vi "LoadConfigFile.vi"(8 "error in":errorcluster, 11 "Model Name":string) -> (0 "error out":errorcluster, 1 "path":path, 2 "ConnectConfig":T1={"IP Address"="", "Port"=102, "Timeout"=5000}, 3 "Data out":T2)   [LabVIEW 2025, in "PLC_Module.lvlib" / "PLC_Module.lvclass"]
uses:
  PLC_Module.lvclass
  PLC_Data_Config.ctl
  PLC_Data.ctl
  PLC_Data_Type.ctl
  PLC_Connect_Config.ctl
  PLC_Config.ctl
  a0ae5e0e-cf4b-4af0-ab00-451458f61aa5.vi
  <vilib>/JDP Science/JSONtext/JSON text to Variant.vi
  <vilib>/JDP Science/JSONtext/LVClass Serializer/JSONtext LVClass Serializer.lvclass
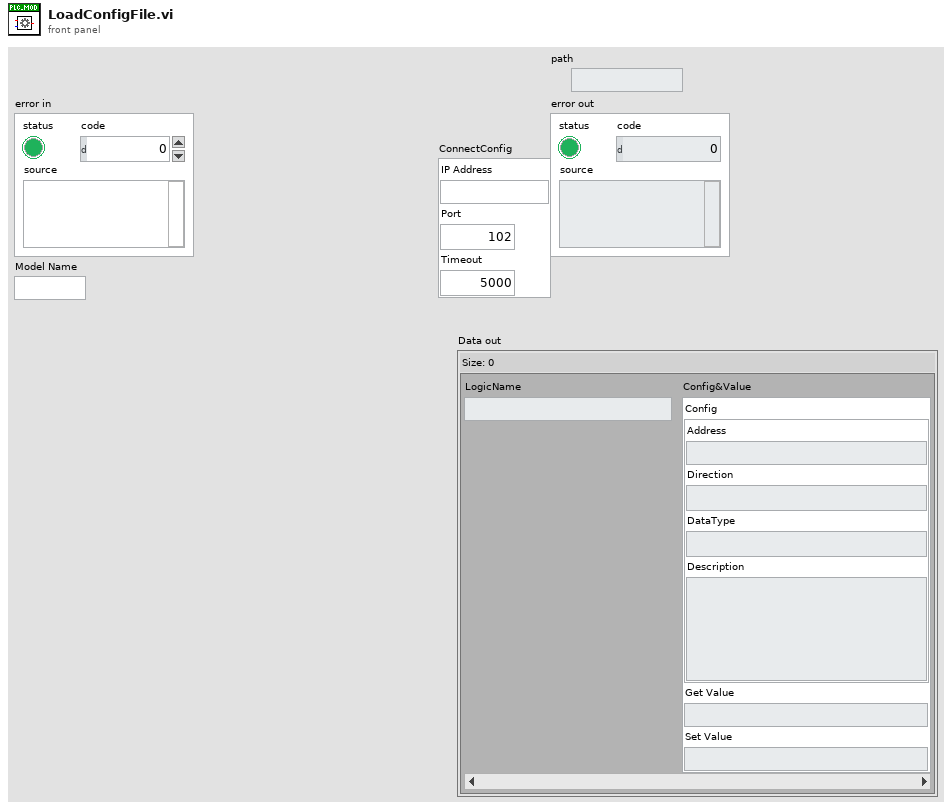
[diagram p1: front panel]
types:
  T1 = typedef "PLC_Module.lvlib/PLC_Module.lvclass/PLC_Connect_Config.ctl" = cluster{"IP Address":string, "Port":u16, "Timeout":i32}
  T2 = typedef "PLC_Module.lvlib/PLC_Module.lvclass/PLC_Data_Config.ctl" = map{string, cluster{"Config":T3, "Get Value":string, "Set Value":string}}
  T3 = typedef "PLC_Module.lvlib/PLC_Module.lvclass/PLC_Data.ctl" = cluster{"Address":string, "Direction":enum16{"PC->PLC", "PLC->PC"}, "DataType":T4, "Description":string}
  T4 = typedef "PLC_Module.lvlib/PLC_Module.lvclass/PLC_Data_Type.ctl" = enum16{"Boolean", "Single Float", "U8", "U32", "U32_Array", "String"}
  T5 = typedef "PLC_Module.lvlib/PLC_Module.lvclass/PLC_Config.ctl" = cluster{"ConnectConfig":T1, "DataConfiguration":T2}
  T6 = enum16{"open", "replace", "create", "open or create", "replace or create", "replace or create with confirmation"}
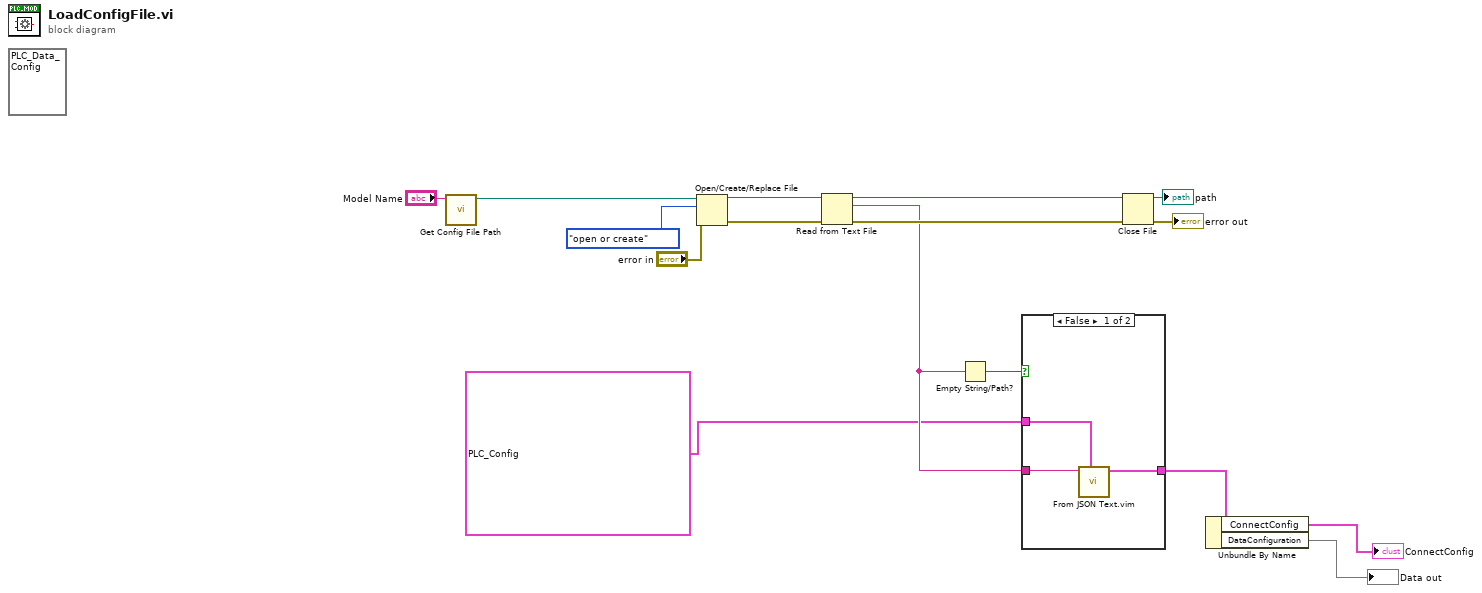
[diagram p0: block diagram]
diagram:
  (unwired) T2 {"PC_AutoManualMode"={"Config"={"Address"="DB6010.703", "Direction"=enum."PC->PLC", "DataType"=enum."U8", "Description"="PC手自动模式"}, "Get Value"="", "Set Value"=""}, "PC_Error"={"Config"={"Address"="DB6010.700[3]", "Direction"=enum."PC->PLC", "DataType"=enum."Boolean", "Description"="错误信息"}, "Get Value"="", "Set Value"=""}, "PC_ErrorCode"={"Config"={"Address"="DB6010.714", "Direction"=enum."PC->PLC", "DataType"=enum."U32", "Description"=""}, "Get Value"="", "Set Value"=""}, "PC_FDBK_1"={"Config"={"Address"="DB6010.704", "Direction"=enum."PC->PLC", "DataType"=enum."U32", "Description"="读取测试流程信号"}, "Get Value"="", "Set Value"=""}, "PC_HeartBeat"={"Config"={"Address"="DB6010.700[0]", "Direction"=enum."PC->PLC", "DataType"=enum."Boolean", "Description"="PC端心跳信号"}, "Get Value"="", "Set Value"=""}, "PC_ProdCode"={"Config"={"Address"="DB6010.750", "Direction"=enum."PC->PLC", "DataType"=enum."U32", "Description"="向PLC发送配方号"}, "Get Value"="", "Set Value"=""}, "PC_ProdName"={"Config"={"Address"="DB6010.720[28]", "Direction"=enum."PC->PLC", "DataType"=enum."String", "Description"="向PLC发送配方名称"}, "Get Value"="", "Set Value"=""}, "PC_Ready"={"Config"={"Address"="DB6010.700[6]", "Direction"=enum."PC->PLC", "DataType"=enum."Boolean", "Description"=""}, "Get Value"="", "Set Value"=""}, "PC_Running"={"Config"={"Address"="DB6010.700[5]", "Direction"=enum."PC->PLC", "DataType"=enum."Boolean", "Description"=""}, "Get Value"="", "Set Value"=""}, "PC_TotleResult"={"Config"={"Address"="DB6012.0", "Direction"=enum."PC->PLC", "DataType"=enum."U32", "Description"="向PLC发送测试总结果"}, "Get Value"="", "Set Value"=""}, "PLC_AutoManualMode"={"Config"={"Address"="DB6010.3", "Direction"=enum."PLC->PC", "DataType"=enum."U8", "Description"="PLC手自动模式"}, "Get Value"="", "Set Value"=""}, "PLC_DMC"={"Config"={"Address"="DB6010.100[48]", "Direction"=enum."PLC->PC", "DataType"=enum."String", "Description"="从PLC读取SN"}, "Get Value"="", "Set Value"=""}, "PLC_HeartBeat"={"Config"={"Address"="DB6010.0[0]", "Direction"=enum."PLC->PC", "DataType"=enum."Boolean", "Description"="PLC端心跳信号"}, "Get Value"="", "Set Value"=""}, "PLC_ProdCode"={"Config"={"Address"="DB6010.70", "Direction"=enum."PLC->PC", "DataType"=enum."U32", "Description"="向PC发送交互信号"}, "Get Value"="", "Set Value"=""}, "PLC_ProdName"={"Config"={"Address"="DB6010.40[28]", "Direction"=enum."PLC->PC", "DataType"=enum."String", "Description"="向PC发送配方名称"}, "Get Value"="", "Set Value"=""}, "PLC_Stop_CMD"={"Config"={"Address"="DB6010.1[7]", "Direction"=enum."PLC->PC", "DataType"=enum."Boolean", "Description"=""}, "Get Value"="", "Set Value"=""}, "PLC_Task1"={"Config"={"Address"="DB6010.4", "Direction"=enum."PLC->PC", "DataType"=enum."U32", "Description"="从PLC读取任务信号"}, "Get Value"="", "Set Value"=""}} ("Data out 2")
  n1 = call "Get Config File Path.vi"("Model Name"="Model Name") -> ("appended path"=w16:path)  [unwired: 10 in]
  n2 = Open/Create/Replace File(file path (use dialog)=w16, error in="error in", operation (0:open)=T6."open or create") -> (refnum out=w14:refnum<file>, error out=w13:errorcluster)  [unwired: 3 in, 1 out]
  n3 = Read from Text File(file (use dialog)=w14, error in=w13) -> (refnum out=w12:refnum<file>, text=w7:string, error out=w11:errorcluster)  [unwired: 2 in, 1 out]
  n4 = Empty String/Path?(string/path=w7) -> (empty?=w6:bool)
  n5 = case shown="False" w6 {
    tunnel: [w19 w20] -> w4
    tunnel: T5 {"ConnectConfig"={"IP Address"="192.168.1.100", "Port"=502, "Timeout"=3000}, "DataConfiguration"={"PC_AutoManualMode"={"Config"={"Address"="DB6010.703", "Direction"=enum."PC->PLC", "DataType"=enum."U8", "Description"="PC手自动模式"}, "Get Value"="0", "Set Value"="0"}, "PC_Error"={"Config"={"Address"="DB6010.700[3]", "Direction"=enum."PC->PLC", "DataType"=enum."Boolean", "Description"="错误信息"}, "Get Value"="false", "Set Value"=""}, "PC_ErrorCode"={"Config"={"Address"="DB6010.714", "Direction"=enum."PC->PLC", "DataType"=enum."U32", "Description"=""}, "Get Value"="0", "Set Value"=""}, "PC_FDBK_1"={"Config"={"Address"="DB6010.704", "Direction"=enum."PC->PLC", "DataType"=enum."U32", "Description"="读取测试流程信号"}, "Get Value"="0", "Set Value"=""}, "PC_HeartBeat"={"Config"={"Address"="DB6010.700[0]", "Direction"=enum."PC->PLC", "DataType"=enum."Boolean", "Description"="PC端心跳信号"}, "Get Value"="true", "Set Value"=""}, "PC_ProdCode"={"Config"={"Address"="DB6010.750", "Direction"=enum."PC->PLC", "DataType"=enum."U32", "Description"="向PLC发送配方号"}, "Get Value"="0", "Set Value"=""}, "PC_ProdName"={"Config"={"Address"="DB6010.720[28]", "Direction"=enum."PC->PLC", "DataType"=enum."String", "Description"="向PLC发送配方名称"}, "Get Value"="\"\"", "Set Value"="\"\""}, "PC_Ready"={"Config"={"Address"="DB6010.700[6]", "Direction"=enum."PC->PLC", "DataType"=enum."Boolean", "Description"=""}, "Get Value"="false", "Set Value"=""}, "PC_Running"={"Config"={"Address"="DB6010.700[5]", "Direction"=enum."PC->PLC", "DataType"=enum."Boolean", "Description"=""}, "Get Value"="false", "Set Value"=""}, "PC_TotleResult"={"Config"={"Address"="DB6012.0", "Direction"=enum."PC->PLC", "DataType"=enum."U32", "Description"="向PLC发送测试总结果"}, "Get Value"="0", "Set Value"=""}, "PLC_AutoManualMode"={"Config"={"Address"="DB6010.3", "Direction"=enum."PLC->PC", "DataType"=enum."U8", "Description"="PLC手自动模式"}, "Get Value"="0", "Set Value"=""}, "PLC_DMC"={"Config"={"Address"="DB6010.100[48]", "Direction"=enum."PLC->PC", "DataType"=enum."String", "Description"="从PLC读取SN"}, "Get Value"="\"\"", "Set Value"=""}, "PLC_HeartBeat"={"Config"={"Address"="DB6010.0[0]", "Direction"=enum."PLC->PC", "DataType"=enum."Boolean", "Description"="PLC端心跳信号"}, "Get Value"="true", "Set Value"=""}, "PLC_ProdCode"={"Config"={"Address"="DB6010.70", "Direction"=enum."PLC->PC", "DataType"=enum."U32", "Description"="向PC发送交互信号"}, "Get Value"="0", "Set Value"=""}, "PLC_ProdName"={"Config"={"Address"="DB6010.40[28]", "Direction"=enum."PLC->PC", "DataType"=enum."String", "Description"="向PC发送配方名称"}, "Get Value"="\"\"", "Set Value"=""}, "PLC_StartTest"={"Config"={"Address"="DB6010.1[1]", "Direction"=enum."PC->PLC", "DataType"=enum."Boolean", "Description"="启动测试流程"}, "Get Value"="false", "Set Value"=""}, "PLC_Stop_CMD"={"Config"={"Address"="DB6010.1[7]", "Direction"=enum."PLC->PC", "DataType"=enum."Boolean", "Description"=""}, "Get Value"="false", "Set Value"=""}, "PLC_Task1"={"Config"={"Address"="DB6010.4", "Direction"=enum."PLC->PC", "DataType"=enum."U32", "Description"="从PLC读取任务信号"}, "Get Value"="0", "Set Value"=""}, "PLC_TerminateProcess"={"Config"={"Address"="DB6010.1[2]", "Direction"=enum."PLC->PC", "DataType"=enum."Boolean", "Description"="终止测试程序，结束PLC模块"}, "Get Value"="false", "Set Value"=""}}} ("PLC_Config") -> [w18 w20]
    tunnel: w7 -> [w17 _]
    frame False {
      n6 = call "From JSON Text.vim"("Data Type and Default Value"=w18, "JSON"=w17) -> ("Data out"=w19:T5)  [unwired: 8 in, 1 out]
    }
    frame True {
    }
  }
  n7 = Close File(refnum=w12, error in=w11) -> (path=→"path":path, error out=→"error out":errorcluster)
  n8 = Unbundle By Name(w4) -> ("ConnectConfig"=→"ConnectConfig":T1, "DataConfiguration"=→"Data out":T2)
